vi "ziExample-HDAWG-Module-AWG.vi"() -> ()   [LabVIEW 2009]
doc: "Control a Zurich instrument device via the LabOne Labview API. \nRequirements: Zurich Instruments UHFLI \nThis example shows how to start a AWG module and measure it with the scope module.\n\n© Zurich Instruments AG, www.zhinst.com"
uses:
  <instrlib>/Zurich Instruments LabOne/Public/Modules/ziTypeModEnum.ctl
  <instrlib>/Zurich Instruments LabOne/Public/Configure/ziSetValueDouble.vi
  <instrlib>/Zurich Instruments LabOne/Public/Modules/ziModSetValueBinary.vi
  <instrlib>/Zurich Instruments LabOne/Public/Modules/ziModSetValueDouble.vi
  <instrlib>/Zurich Instruments LabOne/Zurich Instruments LabOne.lvlib
panel:
  in  "stop":bool
  out "Status":bool
  out "Finish":bool
  in  "AWG":string="// Define an integer constant\nconst N = 4096;\n// Create  Gaussian pulses with length N points,\n// amplitude +1.0, center at N/2, and a width of N/8\nwave gauss = 1.0*gauss(N, N/2, N/8);\n\nplayWave(gauss);\nsetTrigger(1);\nsetTrigger(0);"
  out "Error Out":errorcluster
  in  "Address":string="DEV"
  out "Selected Device":string
  # "ziExample-HDAWG-Module-AWG.vi\nRequirements: HDAWG\nsee block diagram for VI description"
  # "Tested Devices:\n- HDAWG"
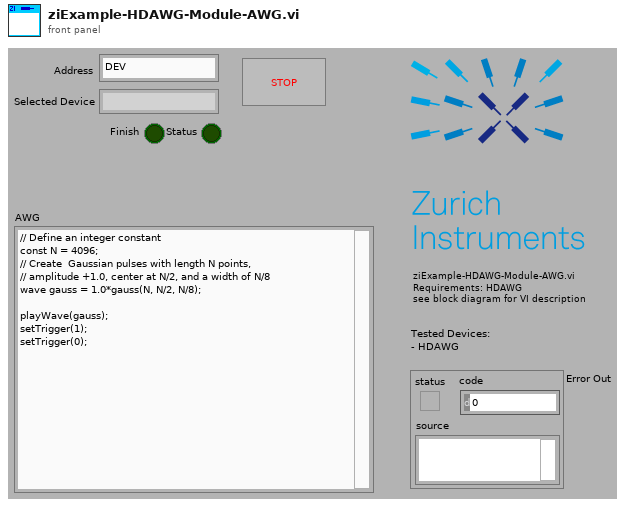
[diagram p1: front panel]
types:
  T1 = typedef "Zurich Instruments LabOne.lvlib/ziTypeModEnum.ctl" = u16
  T2 = typedef "Zurich Instruments LabOne.lvlib/ziTypeHandle.ctl" = cluster{"handleValid":bool, "Conn":u64, "Path Prefix":string, "Handle":u64, "Connected":bool, "Clockbase(s)":dbl}
  T3 = typedef "Zurich Instruments LabOne.lvlib/ziTypeModHandle.ctl" = cluster{"handleValid":bool, "Conn":u64, "ModHandle":u64, "moduleID":string, "Path Prefix":string}
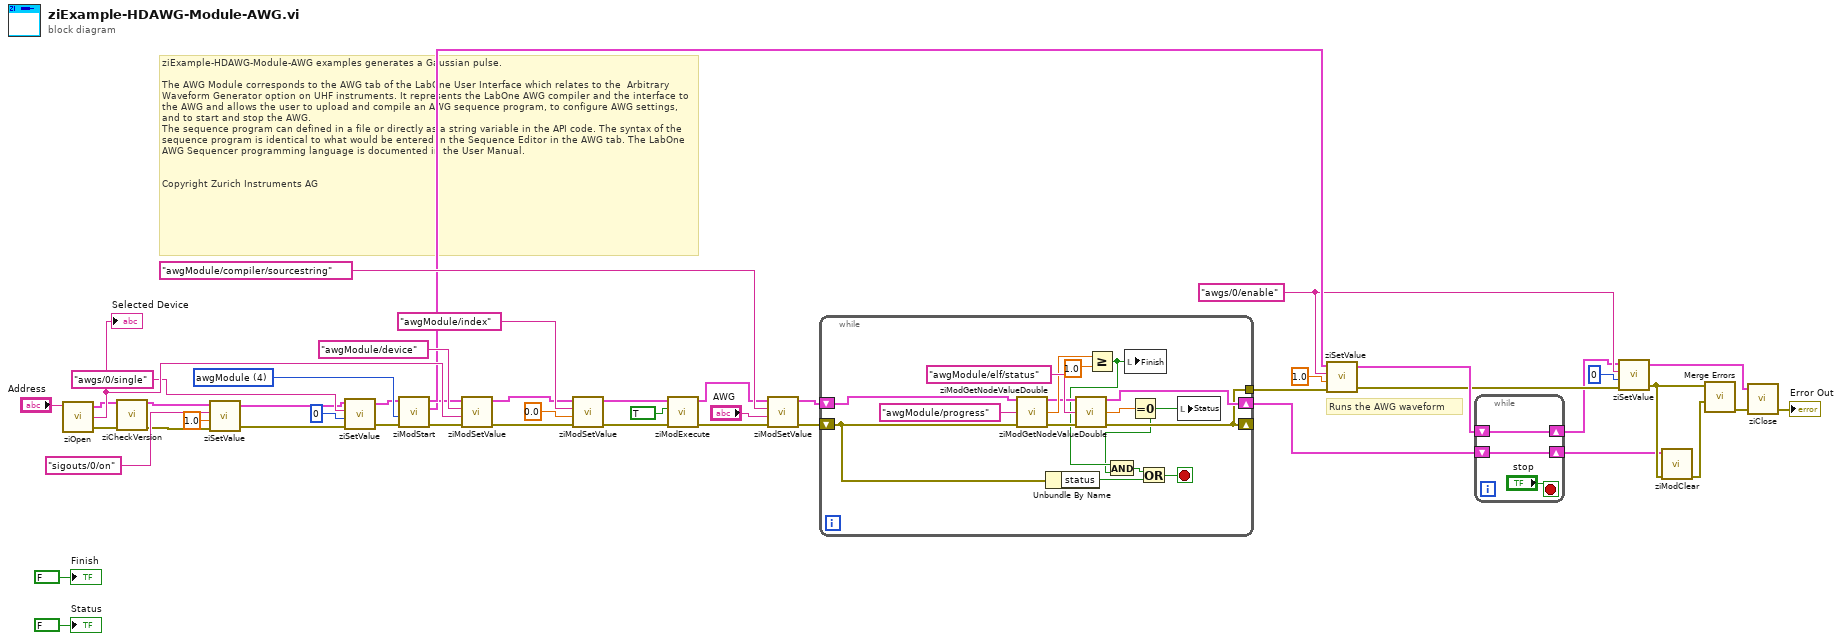
[diagram p0: block diagram]
diagram:
  w38 = T1 4 items=["sweep", "scopeModule", "dataAcquisitionModule", "pidAdvisor", "awgModule", "impedanceModule", "multiDeviceSyncModule", "zoomFFT", "trigger", "deviceSettings", "record"] ("module Id")
  w20 = "awgs/0/enable"
  # "Runs the AWG waveform"
  # "ziExample-HDAWG-Module-AWG examples generates a Gaussian pulse.\n\nThe AWG Module corresponds to the AWG tab of the LabOne User Interface which relates to the  Arbitrary Waveform Generator option on UHF instruments. It represents the LabOne AWG compiler and the interface to the AWG and allows the user to upload and compile an AWG sequence program, to configure AWG settings, and to start and stop the AWG.\nThe sequence program can defined in a file or directly as a string variable in the API code. The syntax of the sequence program is identical to what would be entered in the Sequence Editor in the AWG tab. The LabOne AWG Sequencer programming language is documented in the User Manual.\n\n\nCopyright Zurich Instruments AG"
  n1 = call <instrlib>:"ziOpen.vi"("Address"="Address") -> ("Error Out"=w40:errorcluster, "Selected Device"=w45:string, "HandleOut"=w39:T2)  [unwired: 1 in, 2 out]
  "Selected Device" <- w45
  n2 = call <instrlib>:"ziCheckVersion.vi"("Handle In"=w39, "Error In"=w40) -> ("Handle Out"=w5:T2, "Error Out"=w4:errorcluster)  [unwired: 11 in, 1 out]
  n3 = call-poly <instrlib>:"ziSetValue.vi"("Error In"=w4, "Value"=1.0, "Path"="sigouts/0/on", "Handle In"=w5) -> ("Error Out"=w2:errorcluster, "Handle Out"=w3:T2)  [unwired: 1 in]
  n4 = call-poly <instrlib>:"ziSetValue.vi"("Error In"=w2, "Value"=0, "Path"="awgs/0/single", "Handle In"=w3) -> ("Error Out"=w15:errorcluster, "Handle Out"=w16:T2)  [unwired: 1 in]
  n5 = call <instrlib>:"ziModStart.vi"("Error In"=w15, "module Id"=w38, "Handle In"=w16) -> ("Error Out"=w7:errorcluster, "ModHandle Out"=w12:T3, "Handle Out"=w27:T2)  [unwired: 6 in]
  n6 = call-poly <instrlib>:"ziModSetValue.vi"("Error In"=w7, "Data"=w45, "Path"="awgModule/device", "ModHandle In"=w12) -> ("Error Out"=w8:errorcluster, "ModHandle Out"=w11:T3)  [unwired: 6 in]
  n7 = call-poly <instrlib>:"ziModSetValue.vi"("Error In"=w8, "Value"=0.0, "Path"="awgModule/index", "ModHandle In"=w11) -> ("Error Out"=w9:errorcluster, "ModHandle Out"=w10:T3)  [unwired: 6 in]
  n8 = call <instrlib>:"ziModExecute.vi"("Error In"=w9, "Modal (F)"=TRUE, "ziModHandle In"=w10) -> ("Error Out"=w32:errorcluster, "ziModHandle Out"=w33:T3)  [unwired: 5 in, 1 out]
  n9 = call-poly <instrlib>:"ziModSetValue.vi"("Error In"=w32, "Data"="AWG", "Path"="awgModule/compiler/sourcestring", "ModHandle In"=w33) -> ("Error Out"=w30:errorcluster, "ModHandle Out"=w31:T3)  [unwired: 6 in]
  n10 = while {
    shift-right: [w57] -> w24
    shift-left: w31 -> [w59]
    shift-right: [w51] -> _
    shift-left: w30 -> [w53]
    tunnel: [w51] -> w26
    stop <- w55 stop-if-true
    n11 = call <instrlib>:"ziModGetNodeValueDouble.vi"("ModHandle In"=w59, "Path"="awgModule/progress", "error in"=w53) -> ("ModHandle Out"=w58:T3, "Value"=w61:dbl, "error out"=w56:errorcluster)  [unwired: 10 in]
    n12 = Unbundle By Name(w53) -> ("status"=w52:bool)
    n13 = call <instrlib>:"ziModGetNodeValueDouble.vi"("ModHandle In"=w58, "Path"="awgModule/elf/status", "error in"=w56) -> ("ModHandle Out"=w57:T3, "Value"=w60:dbl, "error out"=w51:errorcluster)  [unwired: 10 in]
    n14 = Greater Or Equal?(x=w61, y=1.0) -> (x >= y?=w50:bool)
    n15 = local write "Finish"(w50) -> ()
    n16 = Equal To 0?(x=w60) -> (x = 0?=w49:bool)
    n17 = And(x=w50, y=w49) -> (x .and. y?=w54:bool)
    n18 = Or(x=w54, y=w52) -> (x .or. y?=w55:bool)
    n19 = local write "Status"(w49) -> ()
  }
  n20 = call-poly <instrlib>:"ziSetValue.vi"("Error In"=w26, "Value"=1.0, "Path"=w20, "Handle In"=w27) -> ("Error Out"=w23:errorcluster, "Handle Out"=w25:T2)  [unwired: 1 in]
  n21 = while {
    shift-right: [w66] -> w19
    shift-left: w24 -> [w66]
    shift-right: [w67] -> w18
    shift-left: w25 -> [w67]
    stop <- "stop" stop-if-true
  }
  n22 = call-poly <instrlib>:"ziSetValue.vi"("Error In"=w23, "Value"=0, "Path"=w20, "Handle In"=w18) -> ("Error Out"=w22:errorcluster, "Handle Out"=w17:T2)  [unwired: 1 in]
  n23 = call <instrlib>:"ziModClear.vi"("Error In"=w22, "ziModHandle In"=w19) -> ("Error Out"=w44:errorcluster)  [unwired: 7 in, 1 out]
  n24 = call <vilib>:"Merge Errors.vi"("error in 3 (no error)"=w44, "error in 1 (no error)"=w22) -> ("error out"=w46:errorcluster)  [unwired: 5 in]
  n25 = call <instrlib>:"ziClose.vi"("Error In"=w46, "Handle In"=w17) -> ("Error Out"=→"Error Out":errorcluster)  [unwired: 2 in, 1 out]
  "Finish" <- FALSE ("Finish")
  "Status" <- FALSE ("Status")
